vi "Timestamp Conversion Single.vi"(9 "timestamp":timestamp) -> (2 "timestamp (ns)":i64)   [LabVIEW 2026, in "synnax_clib.lvlib"]
uses:
  synnax_clib.lvlib
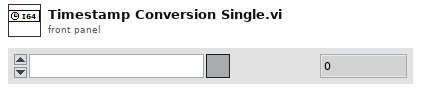
[diagram p1: front panel]
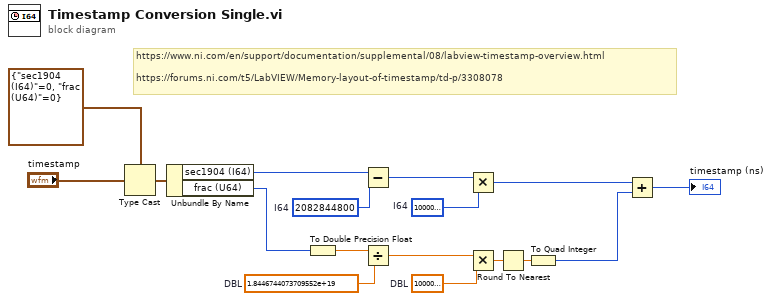
[diagram p0: block diagram]
diagram:
  w7 = 1000000000.0  # DBL
  w9 = 1.8446744073709552e+19  # DBL
  w12 = i64 1000000000  # I64
  w14 = i64 2082844800  # I64
  # "https://www.ni.com/en/support/documentation/supplemental/08/labview-timestamp-overview.html\n\nhttps://forums.ni.com/t5/LabVIEW/Memory-layout-of-timestamp/td-p/3308078"
  n1 = Type Cast(type=cluster{"sec1904 (I64)":i64, "frac (U64)":u64} {"sec1904 (I64)"=0, "frac (U64)"=0}, x="timestamp") -> (*(type *) &x=w16:cluster{"sec1904 (I64)":i64, "frac (U64)":u64})
  n2 = Unbundle By Name(w16) -> ("sec1904 (I64)"=w15:i64, "frac (U64)"=w11:u64)
  n3 = To Double Precision Float(number=w11) -> (double precision float=w10:dbl)
  n4 = Subtract(x=w15, y=w14) -> (x-y=w13:i64)
  n5 = Divide(x=w10, y=w9) -> (x/y=w8:dbl)
  n6 = Multiply(x=w13, y=w12) -> (x*y=w4:i64)
  n7 = Multiply(x=w8, y=w7) -> (x*y=w6:dbl)
  n8 = Round To Nearest(number=w6) -> (nearest integer value=w5:dbl)
  n9 = To Quad Integer(1:w5) -> (0:w3:i64)
  n10 = Add(x=w4, y=w3) -> (x+y=→"timestamp (ns)":i64)
